vi "Thermal Chamber Response Simulator_Init-UTF-Teardown.vi"() -> (1 "Ramp Rate (deg C per second)":dbl, 2 "Temperature Set Point (deg C)":dbl, 3 "Actual Temperature":dbl, 4 "Application Exit":bool, 6 "Heater State":bool)   [LabVIEW 2018]
uses:
  Libraries/Thermal Chamber Response Simulator/Thermal Chamber Response Simulator.lvlib
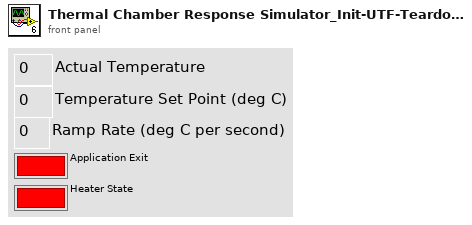
[diagram p1: front panel]
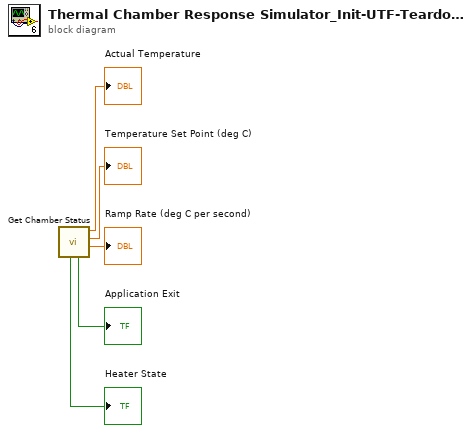
[diagram p0: block diagram]
diagram:
  n1 = call "Get Chamber Status.vi"() -> ("Ramp Rate (deg C / second)"=→"Ramp Rate (deg C per second)":dbl, "Temperature Set Point (deg C)"=→"Temperature Set Point (deg C)":dbl, "Actual Temperature"=→"Actual Temperature":dbl, "Application Exit"=→"Application Exit":bool, "Heater State"=→"Heater State":bool)  [unwired: 6 in, 1 out]
